vi "File Reference Warning.vi"(8 "error in (no error)":errorcluster, 11 "Message (\"\")":string="Spartan cannot find the data file(s) that is(are) being referenced by this test step.\n\nPlease select one of the following options:\n\n    Ignore - continue without the referenced articles being applied\n    Abort - abort this test step\n    Abort All - abort this and all remaining test steps in the sequence") -> (0 "error out":errorcluster, 2 "Choice":i32, 3 "Command":string)   [LabVIEW 2011]
panel:
  in  "Abort All":bool
  in  "Abort":bool
  in  "Ignore":bool
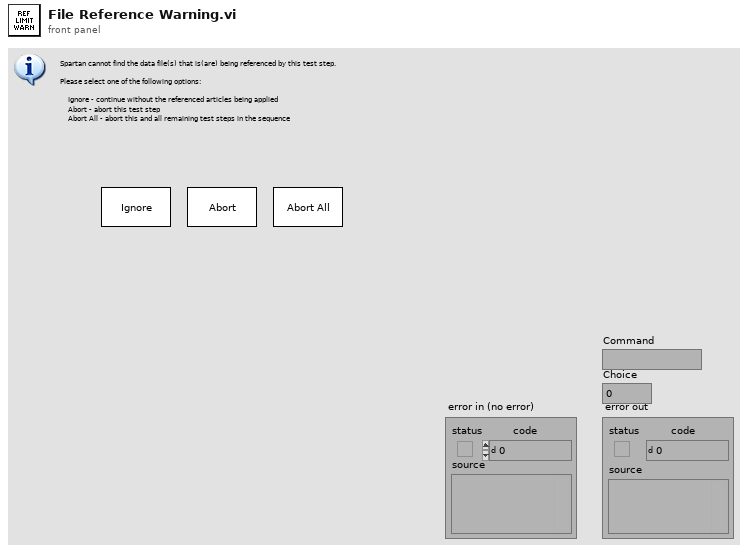
[diagram p1: front panel]
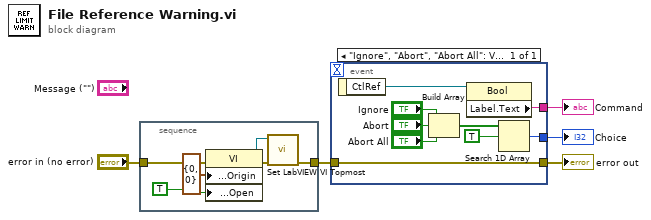
[diagram p0: block diagram]
diagram:
  n1 = stacked-sequence {
    tunnel: "error in (no error)" -> [w11]
    tunnel: [w8] -> w3
    frame #0 {
      n2 = property on="Property Node" class="VI"(error in=w11, "Front Panel Window:Origin"=cluster{"Horizontal":i16, "Vertical":i16} {"Horizontal"=0, "Vertical"=0}, "Front Panel Window:Open"=TRUE) -> (reference out=w7:refnum<vi>, error out=w9:errorcluster)  [unwired: 1 in]
      n3 = call "Set LabVIEW VI Topmost.vi"("error in (no error)"=w9, "VI Refnum (null)"=w7) -> ("error out"=w8:errorcluster)  [unwired: 7 in, 2 out]
    }
  }
  n4 = event shown="[0] \"Ignore\", \"Abort\", \"Abort All\": Value Change" {
    selector: _ -> [_]
    dyn-events: _ -> [_]
    timeout: _ -> [_]
    tunnel: w3 -> [w20]
    tunnel: [w20] -> w5
    tunnel: [w14] -> w2
    tunnel: [w12] -> w1
    event "Ignore", "Abort", "Abort All": Value Change {
      n5 = event-data() -> ("CtlRef"=w13:refnum<vi>)  [unwired: 1 out]
      n6 = Build Array("Ignore", "Abort", "Abort All") -> (w16:bool[])
      n7 = property class="Bool"(reference=w13) -> ("Label.Text"=w12:string)  [unwired: 1 in, 2 out]
      n8 = Search 1D Array(1D array=w16, element=TRUE) -> (index of element=w14:i32)  [unwired: 1 out]
    }
  }
  "error out" <- w5
  "Choice" <- w2
  "Command" <- w1
